vi "Lookup Error Codes.vi"(8 "error in (no error)":errorcluster, 11 "Node Ptr":u64) -> (0 "error out":errorcluster, 2 "Error Codes":cluster{"Code":i32, "String":string}[](array[cluster]), 3 "Node Ptr out":u64)   [LabVIEW 2019, in "Instrument Addon Shared.lvlib"]
uses:
  Instrument Addon Shared.lvlib
  Types/FG Control.ctl
  Constants.vi
  <vilib>/NI/NI VeriStand Advanced SysDef API/SysDef API/SysDef.Property.Get.vi
  <vilib>/NI/NI VeriStand Advanced SysDef API/_SubVIs/SysDef.Property.Get.String.vi
  <vilib>/NI/NI VeriStand Advanced SysDef API/SysDef API/SysDef.Property.Set.vi
  <vilib>/NI/NI VeriStand Advanced SysDef API/_SubVIs/SysDef.Property.Set.String.vi
  <vilib>/Utility/LVClass/Get LV Class Default Value.vi
  Support Libraries/Protocols.lvlibp/Protocol Parent/Protocol Parent.lvclass
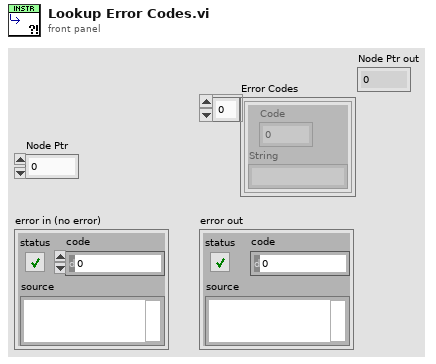
[diagram p1: front panel]
types:
  T1 = typedef "Instrument Addon Shared.lvlib/FG Control.ctl" = enum16{"Get", "Set"}
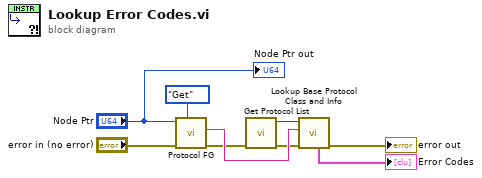
[diagram p0: block diagram]
diagram:
  n1 = call "Protocol FG.vi"("Action"=FG_Control."Get", "error in (no error)"="error in (no error)", "Device Item Ref in"="Node Ptr") -> ("error out"=w6:errorcluster, "Protocol out"=w7:string)  [unwired: 6 in, 1 out]
  n2 = call "Get Protocol List.vi"("error in (no error)"=w6) -> ("error out"=w5:errorcluster, "Class Lookup"=w4:variant)  [unwired: 9 in]
  n3 = call "Lookup Base Protocol Class and Info.vi"("error in (no error)"=w5, "Protocol in"=w7, "Class Lookup"=w4) -> ("error out"=→"error out":errorcluster, "Error Codes"=→"Error Codes":cluster{"Code":i32, "String":string}[])  [unwired: 4 in, 3 out]
  "Node Ptr out" <- "Node Ptr"
